vi "Cam Live Location.vi"() -> ()   [LabVIEW 2013]
doc: "The Low-Level Grab Raw Data VI acquires images continuously using low-level acquisition VIs. This VI demonstrates how to acquire raw data from the camera. A grab is appropriate for high-speed applications in which you need to process only one image at a time."
uses:
  <vilib>/userdefined/High Color/IMAQdx.ctl
  <vilib>/vision/driver/IMAQdx.llb/IMAQdx Buffer Number Mode.ctl
  <vilib>/vision/driver/NI_Vision_Acquisition_Software.lvlib
  <vilib>/vision/NI_Vision_Development_Module.lvlib
panel:
  in  "Camera":T1
  in  "Minimum Match Score":sgl=200.0
  out "Number of Matches":i32
  out "x-y":u32
  out "Tube":u8[][](graph)
  out "Bird":u8[][](graph)
  out "XY Graph":cluster{sgl[], sgl[]}(graph)
  out "y":sgl(graph)
  out "x":sgl(graph)
  out "Image":T2(plugin-control)
  in  "Stop":bool
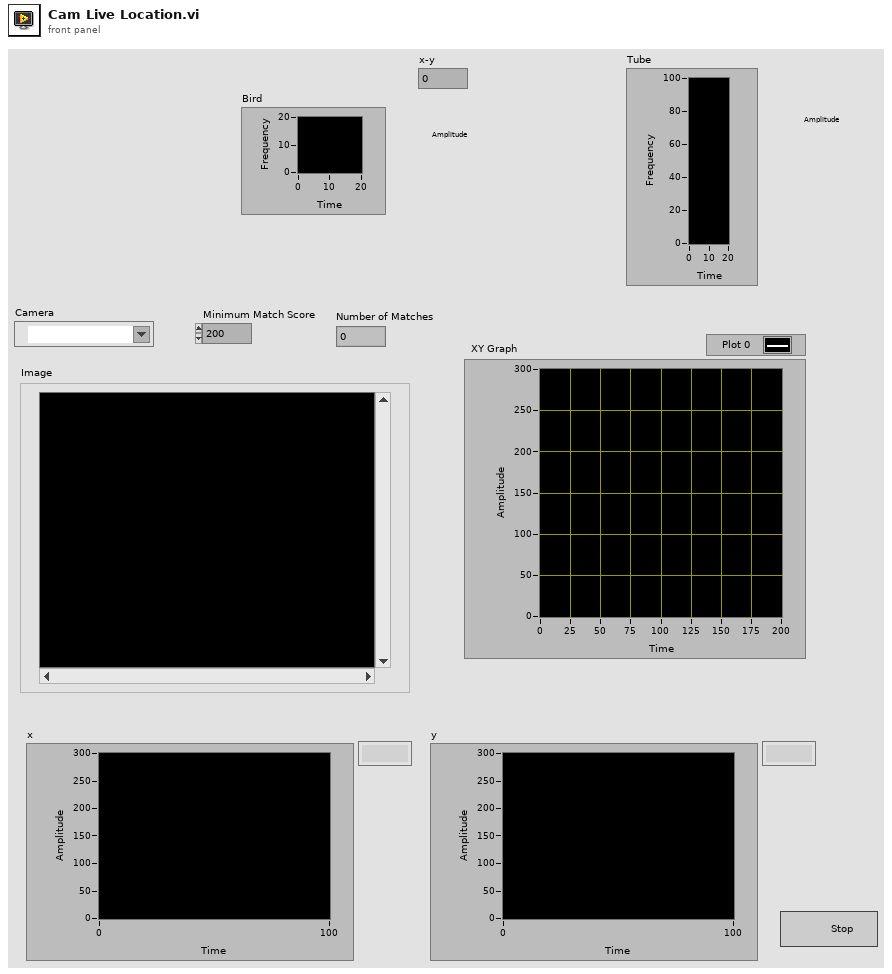
[diagram p1: front panel]
types:
  T1 = typedef "IMAQdx.ctl" = refnum<k21>
  T2 = typedef "IMAQ Image.ctl" = refnum<image>
  T3 = typedef "NI_Vision_Acquisition_Software.lvlib/IMAQdx Buffer Number Mode.ctl" = enum32{"Next", "Last", "Buffer Number"}
  T4 = typedef "Image Type" = u32
  T5 = cluster{"Position":cluster{"x":sgl, "y":sgl}, "Angle":sgl, "Scale":sgl, "Score":sgl, "Bounding Box":cluster{"x":sgl, "y":sgl}[]}[]
  T6 = cluster{"Position":cluster{"x":sgl, "y":sgl}, "Angle":sgl, "Scale":sgl, "Score":sgl, "Bounding Box":cluster{"x":sgl, "y":sgl}[]}
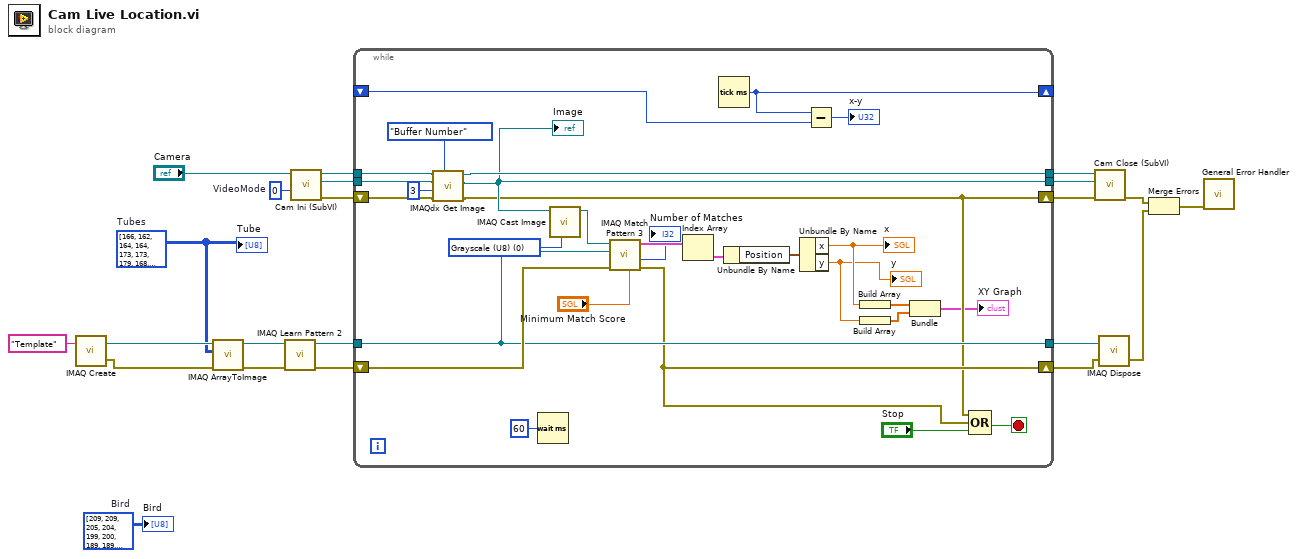
[diagram p0: block diagram]
diagram:
  w2 = u8[][] [[166, 162, 164, 164, 173, 173, 179, 168, 212, 217, 232, 233, 234, 244, 255, 255, 255, 255, 255, 255, 255, 255, 255, 255, 255, 255, 255, 255, 255, 255, 243, 230, 223, 219, 217, 216, 218, 218, 219, 221, 218, 218, 218, 218, 221, 222, 220, 220, 217, 217, 222, 223, 218, 219, 223, 223, 217, 215, 220, 221, 218, 213, 227, 227, 218, 221, 215, 212, 217, 220, 213, 212, 212, 213, 215, 216, 215, 216, 221, 221, 215, 213, 214, 213, 206, 204, 209, 209, 208, 209, 205, 208, 208, 206, 206, 205, 211, 215, 207, 207], [146, 143, 144, 143, 143, 141, 154, 143, 205, 207, 222, 217, 215, 224, 228, 239, 255, 255, 255, 255, 255, 255, 255, 255, 255, 255, 255, 255, 255, 255, 230, 219, 217, 217, 215, 213, 220, 220, 221, 223, 219, 220, 222, 222, 221, 222, 219, 218, 228, 228, 223, 226, 214, 216, 220, 220, 214, 213, 218, 218, 220, 220, 216, 219, 218, 222, 215, 215, 216, 217, 217, 221, 210, 209, 217, 219, 220, 220, 215, 217, 218, 216, 206, 204, 201, 202, 201, 201, 201, 197, 200, 199, 200, 197, 199, 201, 203, 204, 209, 210], [132, 132, 130, 128, 130, 127, 138, 125, 186, 186, 193, 190, 188, 206, 205, 220, 221, 225, 231, 230, 225, 225, 229, 221, 235, 235, 255, 255, 255, 249, 225, 221, 213, 215, 213, 212, 217, 216, 212, 215, 225, 221, 217, 217, 221, 223, 215, 217, 220, 219, 220, 220, 218, 218, 217, 215, 223, 223, 224, 223, 214, 214, 215, 215, 221, 225, 222, 226, 219, 220, 216, 218, 216, 217, 216, 217, 216, 217, 213, 213, 209, 202, 201, 203, 181, 181, 183, 183, 180, 179, 180, 179, 179, 173, 177, 174, 193, 195, 191, 189], [122, 120, 121, 120, 122, 118, 127, 121, 156, 157, 153, 150, 143, 164, 178, 201, 198, 197, 203, 203, 201, 200, 196, 182, 212, 207, 255, 255, 254, 241, 223, 221, 215, 215, 218, 220, 215, 212, 214, 214, 215, 215, 220, 219, 221, 221, 227, 230, 219, 220, 217, 219, 221, 218, 220, 218, 219, 220, 220, 220, 217, 217, 217, 218, 220, 219, 217, 218, 216, 216, 220, 219, 218, 220, 213, 214, 214, 217, 219, 222, 211, 209, 189, 198, 169, 169, 171, 176, 170, 171, 172, 179, 171, 145, 143, 134, 159, 165, 183, 186], [110, 110, 115, 111, 112, 112, 111, 105, 128, 123, 123, 113, 110, 159, 163, 187, 198, 201, 196, 194, 200, 199, 185, 159, 188, 173, 250, 251, 249, 236, 223, 219, 222, 222, 221, 222, 217, 217, 217, 216, 215, 215, 223, 225, 215, 212, 217, 217, 224, 226, 214, 213, 216, 213, 214, 216, 214, 210, 218, 218, 219, 218, 219, 215, 219, 219, 221, 220, 221, 220, 218, 218, 211, 213, 213, 212, 221, 221, 221, 221, 206, 204, 177, 195, 170, 174, 166, 176, 181, 184, 175, 180, 163, 147, 125, 102, 133, 142, 145, 145], [109, 111, 109, 109, 111, 111, 117, 101, 111, 108, 99, 82, 104, 128, 166, 199, 198, 198, 198, 198, 199, 198, 187, 163, 185, 165, 246, 251, 255, 240, 222, 218, 219, 218, 222, 222, 220, 219, 220, 220, 217, 216, 219, 219, 221, 221, 220, 220, 220, 220, 222, 220, 221, 218, 222, 221, 221, 222, 215, 210, 214, 214, 213, 210, 213, 213, 215, 215, 218, 220, 213, 215, 210, 211, 216, 216, 213, 216, 217, 217, 201, 202, 188, 198, 172, 196, 183, 185, 186, 183, 190, 183, 177, 149, 116, 81, 110, 122, 123, 125], [132, 130, 125, 125, 128, 125, 130, 127, 120, 106, 83, 72, 101, 143, 174, 212, 202, 202, 207, 206, 209, 208, 197, 154, 187, 162, 255, 255, 255, 251, 238, 231, 222, 223, 218, 221, 215, 217, 215, 214, 221, 221, 216, 217, 222, 221, 220, 216, 218, 218, 212, 215, 222, 221, 219, 219, 218, 218, 218, 218, 214, 217, 216, 216, 217, 219, 210, 215, 214, 217, 212, 211, 214, 214, 218, 217, 217, 220, 219, 221, 208, 206, 180, 219, 194, 209, 194, 199, 194, 194, 192, 192, 177, 150, 115, 74, 96, 116, 119, 124], [145, 145, 143, 140, 143, 138, 137, 137, 137, 112, 94, 60, 91, 130, 175, 203, 219, 219, 213, 213, 219, 219, 207, 167, 186, 159, 255, 255, 255, 255, 255, 243, 218, 217, 210, 211, 217, 221, 217, 214, 220, 219, 214, 213, 218, 220, 217, 214, 219, 216, 217, 214, 220, 220, 216, 215, 216, 216, 216, 215, 221, 221, 216, 215, 214, 213, 216, 212, 220, 222, 215, 216, 217, 217, 215, 218, 215, 215, 213, 212, 207, 207, 184, 217, 198, 207, 200, 200, 206, 207, 208, 208, 185, 141, 111, 70, 88, 116, 126, 125], [155, 156, 150, 150, 157, 156, 153, 154, 147, 129, 101, 74, 104, 146, 184, 203, 211, 211, 213, 213, 217, 217, 210, 170, 189, 160, 254, 255, 255, 255, 255, 255, 232, 221, 219, 219, 220, 221, 216, 217, 218, 218, 221, 222, 213, 212, 217, 219, 219, 218, 220, 219, 217, 217, 219, 221, 217, 216, 220, 219, 215, 214, 218, 218, 216, 217, 212, 211, 213, 214, 214, 212, 214, 214, 213, 217, 216, 217, 220, 221, 202, 199, 184, 212, 199, 208, 203, 202, 205, 205, 211, 210, 177, 140, 107, 70, 99, 126, 130, 140], [167, 167, 166, 164, 167, 168, 168, 170, 167, 136, 112, 72, 96, 129, 166, 199, 211, 211, 211, 211, 209, 209, 204, 179, 188, 159, 255, 255, 255, 255, 255, 255, 238, 228, 223, 221, 223, 220, 219, 217, 219, 219, 217, 217, 213, 214, 215, 216, 221, 222, 216, 216, 218, 214, 221, 221, 214, 214, 218, 218, 214, 212, 220, 219, 210, 208, 215, 215, 215, 215, 215, 214, 212, 213, 209, 211, 215, 215, 219, 221, 207, 204, 188, 224, 196, 207, 207, 207, 200, 201, 204, 204, 190, 141, 107, 77, 99, 129, 148, 159], [182, 183, 182, 181, 176, 176, 178, 177, 169, 152, 120, 90, 103, 137, 171, 194, 194, 194, 196, 197, 201, 200, 199, 158, 190, 163, 255, 255, 255, 255, 255, 255, 255, 238, 220, 217, 220, 221, 218, 221, 217, 219, 217, 217, 216, 215, 219, 215, 218, 218, 222, 222, 221, 219, 218, 218, 216, 216, 219, 219, 216, 215, 210, 212, 211, 211, 212, 210, 216, 214, 215, 217, 216, 216, 214, 217, 215, 215, 218, 214, 203, 215, 190, 221, 203, 209, 200, 200, 206, 206, 201, 200, 178, 139, 100, 74, 117, 151, 160, 167], [184, 187, 193, 193, 187, 187, 189, 189, 181, 160, 134, 79, 108, 140, 161, 187, 189, 189, 185, 185, 192, 193, 191, 159, 192, 166, 255, 255, 255, 255, 255, 255, 255, 246, 226, 221, 214, 215, 223, 223, 215, 214, 221, 223, 212, 211, 214, 215, 213, 212, 216, 217, 219, 221, 215, 213, 215, 213, 216, 219, 215, 214, 215, 216, 217, 216, 221, 220, 214, 215, 208, 209, 216, 215, 212, 215, 208, 209, 215, 214, 206, 215, 185, 223, 195, 202, 189, 189, 184, 185, 187, 184, 166, 129, 96, 76, 124, 162, 172, 181], [196, 197, 201, 201, 202, 202, 202, 202, 193, 166, 136, 88, 96, 135, 151, 175, 180, 182, 184, 185, 175, 177, 182, 150, 182, 154, 255, 255, 255, 255, 255, 255, 255, 255, 236, 229, 220, 221, 220, 221, 217, 217, 213, 211, 222, 223, 219, 219, 212, 213, 219, 218, 219, 222, 221, 219, 218, 219, 219, 219, 221, 222, 221, 218, 214, 215, 212, 211, 216, 216, 215, 213, 215, 215, 217, 217, 213, 217, 218, 215, 200, 208, 189, 214, 191, 196, 183, 183, 178, 178, 176, 172, 157, 119, 99, 71, 130, 170, 180, 191], [196, 196, 202, 202, 204, 204, 204, 204, 196, 167, 135, 80, 98, 135, 146, 172, 171, 173, 169, 171, 175, 177, 170, 147, 179, 148, 255, 255, 255, 255, 255, 255, 255, 255, 236, 223, 217, 217, 225, 225, 212, 215, 219, 218, 213, 212, 219, 218, 215, 215, 218, 219, 214, 214, 217, 219, 214, 217, 216, 214, 219, 220, 215, 216, 215, 215, 213, 216, 214, 215, 213, 212, 214, 215, 209, 209, 219, 220, 213, 211, 201, 207, 186, 211, 185, 187, 173, 173, 179, 177, 170, 171, 159, 118, 92, 60, 132, 167, 182, 191], [188, 189, 198, 198, 206, 206, 194, 194, 183, 159, 124, 72, 91, 128, 146, 169, 160, 162, 160, 160, 160, 163, 167, 133, 180, 156, 255, 255, 255, 255, 255, 255, 255, 255, 243, 231, 217, 215, 215, 215, 219, 219, 215, 215, 217, 217, 216, 215, 220, 221, 214, 214, 219, 219, 214, 215, 215, 215, 215, 214, 218, 215, 217, 218, 211, 211, 216, 219, 212, 213, 216, 217, 214, 214, 213, 211, 217, 215, 208, 205, 198, 201, 183, 203, 176, 181, 164, 163, 166, 166, 160, 159, 138, 105, 89, 61, 131, 173, 187, 195]]  # Tubes
  w3 = u8[][] [[209, 209, 205, 204, 199, 200, 189, 189, 196, 196, 207, 209, 200, 200, 206, 208, 204, 203, 207, 208], [210, 211, 203, 205, 199, 206, 199, 188, 185, 176, 183, 189, 195, 196, 202, 202, 204, 203, 204, 205], [204, 207, 209, 217, 205, 226, 206, 203, 173, 166, 156, 148, 175, 172, 194, 193, 201, 202, 202, 199], [197, 205, 203, 224, 225, 244, 255, 230, 187, 160, 136, 135, 154, 150, 183, 181, 194, 193, 204, 202], [198, 205, 202, 215, 233, 255, 255, 255, 198, 173, 134, 129, 151, 137, 171, 161, 188, 189, 203, 202], [191, 199, 190, 196, 218, 245, 255, 255, 204, 187, 141, 136, 137, 123, 160, 151, 182, 179, 198, 198], [180, 187, 170, 178, 175, 211, 224, 218, 184, 172, 131, 127, 131, 119, 149, 136, 172, 164, 189, 190], [177, 183, 155, 163, 157, 178, 183, 190, 164, 162, 118, 120, 125, 114, 145, 126, 173, 161, 189, 189], [170, 179, 138, 148, 122, 131, 126, 133, 119, 123, 109, 109, 122, 108, 141, 118, 159, 142, 192, 188], [175, 179, 132, 142, 107, 115, 94, 102, 106, 115, 115, 111, 130, 115, 153, 135, 163, 157, 185, 185], [177, 185, 135, 144, 108, 115, 101, 113, 125, 131, 145, 142, 170, 161, 178, 162, 180, 168, 191, 188], [172, 178, 141, 145, 99, 110, 110, 118, 156, 166, 190, 199, 217, 215, 226, 208, 207, 184, 196, 189], [179, 181, 145, 150, 113, 120, 129, 149, 188, 203, 241, 249, 255, 255, 249, 235, 213, 199, 200, 191], [189, 190, 148, 146, 125, 138, 146, 166, 200, 222, 255, 255, 255, 255, 251, 232, 209, 193, 196, 190], [195, 194, 165, 164, 131, 152, 148, 156, 204, 214, 243, 252, 253, 244, 236, 209, 207, 194, 197, 196], [195, 192, 163, 164, 136, 155, 141, 165, 188, 190, 214, 228, 220, 214, 215, 185, 198, 182, 203, 201], [194, 192, 172, 173, 135, 147, 141, 144, 164, 169, 189, 187, 201, 199, 188, 179, 196, 188, 208, 205], [195, 193, 170, 171, 138, 143, 132, 131, 138, 143, 172, 169, 182, 176, 191, 183, 199, 197, 209, 209], [203, 203, 184, 183, 145, 143, 129, 122, 130, 134, 137, 144, 171, 169, 192, 191, 203, 203, 213, 217], [204, 204, 199, 198, 169, 169, 160, 157, 157, 157, 164, 170, 186, 190, 207, 207, 209, 211, 209, 207]]  # Bird
  w4 = u32 0  # VideoMode
  n1 = call "IMAQ Create"("Image Name"="Template") -> ("New Image"=w15:T2, "error out"=w13:errorcluster)  [unwired: 4 in]
  n2 = call "IMAQ ArrayToImage"("error in (no error)"=w13, "Image Pixels (U8)"=w2, "Image"=w15) -> ("error out"=w5:errorcluster, "Image Out"=w14:T2)  [unwired: 7 in]
  n3 = call "IMAQ Learn Pattern 2"("error in (no error)"=w5, "Image"=w14) -> ("error out"=w10:errorcluster, "Template Image Out"=w12:T2)  [unwired: 8 in]
  n4 = call "Cam Ini (SubVI).vi"("VideoMode"=w4, "Camera"="Camera") -> ("error out"=w22:errorcluster, "Image Ref"=w19:T2, "Cam Ref"=w21:T1)  [unwired: 7 in]
  n5 = while {
    tunnel: [w46] -> w18
    tunnel: w21 -> [w49]
    tunnel: w19 -> [w48]
    tunnel: [w38] -> w17
    tunnel: w12 -> [w39]
    tunnel: [w39] -> w11
    shift-right: [w34] -> w9
    shift-left: w10 -> [w40]
    shift-right: [w33] -> w20
    shift-left: w22 -> [w47]
    shift-right: [w27] -> _
    shift-left: _ -> [w26]
    stop <- w35 stop-if-true
    w36 = T4 0 items=["Grayscale (U8)", "Grayscale (I16)", "Grayscale (SGL)", "Complex (CSG)", "RGB (U32)", "HSL (U32)", "RGB (U64)", "Grayscale (U16)"] ("Image Type")
    n6 = call <vilib>:"IMAQdx Get Image.vi"("Buffer Number Mode (Next)"=IMAQdx_Buffer_Number_Mode."Buffer Number", "error in"=w47, "Buffer Number In"=u32 3, "Image In"=w48, "Session In"=w49) -> ("error out"=w33:errorcluster, "Image Out"=w38:T2, "Session Out"=w46:T1)  [unwired: 3 in, 1 out]
    "Image" <- w38
    n7 = Wait (ms)(milliseconds to wait=u32 60) -> ()  [unwired: 1 out]
    n8 = call "IMAQ Cast Image"("Image Type"=w36, "Image Src"=w38) -> ("Image Dst Out"=w37:T2)  [unwired: 8 in, 1 out]
    n9 = call "IMAQ Match Pattern 3"("Minimum Match Score"="Minimum Match Score", "error in (no error)"=w40, "Template Image"=w39, "Image"=w37) -> ("error out"=w34:errorcluster, "Number of Matches"=→"Number of Matches":i32, "Matches"=w41:T5)  [unwired: 5 in]
    n10 = Index Array(array=w41) -> (element=w42:T6)  [unwired: 1 in]
    n11 = Tick Count (ms)() -> (millisecond timer value=w27:u32)
    n12 = Unbundle By Name(w42) -> ("Position"=w43:cluster{"x":sgl, "y":sgl})
    n13 = Unbundle By Name(w43) -> ("x"=w32:sgl, "y"=w28:sgl)
    "x" <- w32
    "y" <- w28
    n14 = Subtract(x=w27, y=w26) -> (x-y=→"x-y":u32)
    n15 = Build Array(w32) -> (w31:sgl[])
    n16 = Build Array(w28) -> (w29:sgl[])
    n17 = Bundle(w31, w29) -> (→"XY Graph":cluster{sgl[], sgl[]})  [unwired: 1 in]
    n18 = Compound Arithmetic op=OR(w33, w34, "Stop") -> (w35:bool)
  }
  n19 = call "Cam Close (SubVI).vi"("error in (no error)"=w20, 10:"Refnum in"=w17, 11:"Refnum in"=w18) -> ("error out"=w8:errorcluster)  [unwired: 8 in]
  n20 = call "IMAQ Dispose"("Image"=w11, "error in (no error)"=w9) -> ("error out"=w7:errorcluster)  [unwired: 4 in]
  n21 = Merge Errors(w8, w7) -> (w6:errorcluster)
  n22 = call <vilib>:"General Error Handler.vi"("error in (no error)"=w6) -> ()  [unwired: 1 in, 14 out]
  "Bird" <- w3
  "Tube" <- w2
